vi "VRMSAcqSubVI.vi"(8 "error in (no error)":errorcluster, 11 "Data Cluster in":T1) -> (0 "error out":errorcluster, 2 "RMS value":dbl format="%0.2p", 3 "Data Cluster out":T1)   [LabVIEW 2017]
uses:
  Controls/ShiftRegisterCluster.ctl
  <vilib>/DAQmx/read.llb/DAQmx Read (Analog Wfm 1Chan NSamp).vi
  <vilib>/DAQmx/miscellaneous.llb/DAQmx Fill In Error Info.vi
  <vilib>/measure/madcrms.llb/Basic Averaged DC-RMS for 1 Chan.vi
  <vilib>/measure/NI_MAPro.lvlib
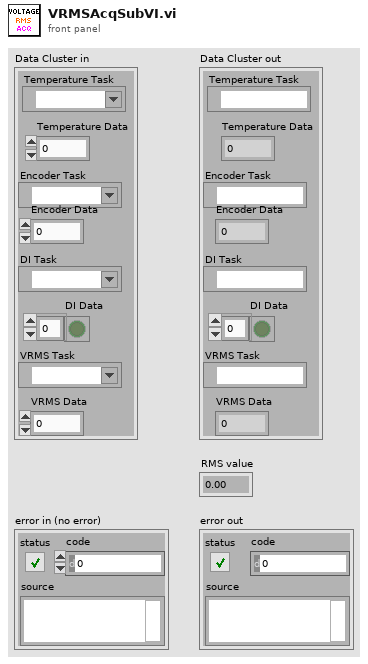
[diagram p1: front panel]
types:
  T1 = typedef "ShiftRegisterCluster.ctl" = cluster{"Temperature Task":refnum<k21>, "Temperature Data":dbl, "Encoder Task":refnum<k21>, "Encoder Data":dbl, "DI Task":refnum<k21>, "DI Data":bool[], "VRMS Task":refnum<k21>, "VRMS Data":dbl}
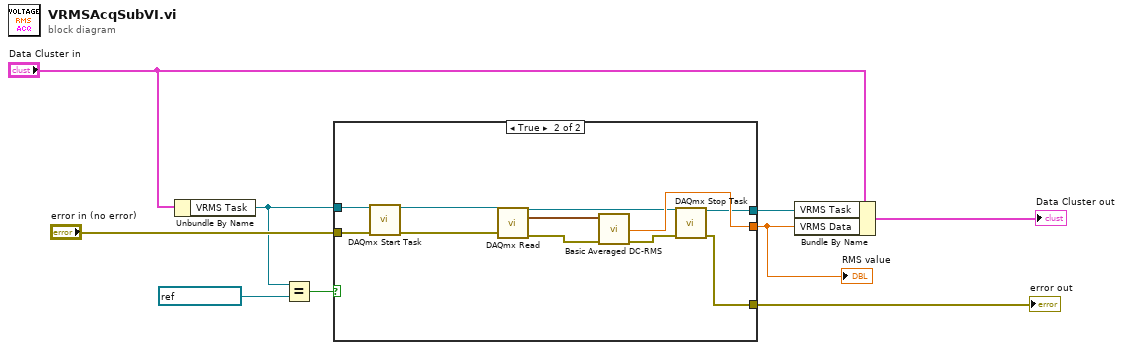
[diagram p0: block diagram]
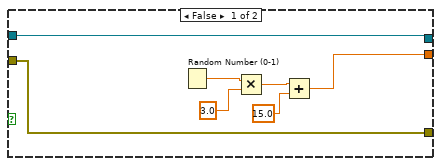
[diagram p2: hidden frame]
diagram:
  n1 = Unbundle By Name("Data Cluster in") -> ("VRMS Task"=w3:refnum<k21>)
  n2 = Equal?(x=w3, y=refnum<k21> "VRMSTask" ("DAQmx Task Name")) -> (x = y?=w1:bool)
  n3 = case shown="True" w1 {
    tunnel: [w11 w27] -> w9
    tunnel: [w16 w23] -> w7
    tunnel: [w10 w22] -> w5
    tunnel: "error in (no error)" -> [w10 w18]
    tunnel: w3 -> [w16 w17]
    frame False {
      n4 = Random Number (0-1)() -> (number: 0 to 1=w15:dbl)
      n5 = Multiply(x=w15, y=3.0) -> (x*y=w13:dbl)
      n6 = Add(x=w13, y=15.0) -> (x+y=w11:dbl)
    }
    frame True {
      n7 = call <vilib>:"DAQmx Start Task.vi"("task/channels in"=w17, "error in"=w18) -> ("task out"=w19:refnum<k21>, "error out"=w20:errorcluster)  [unwired: 12 in]
      n8 = call-poly <vilib>:"DAQmx Read.vi"("task/channels in"=w19, "error in"=w20) -> ("task out"=w21:refnum<k21>, "data"=w24:waveform(dbl), "error out"=w25:errorcluster)  [unwired: 11 in]
      n9 = call-poly <vilib>:"Basic Averaged DC-RMS.vi"("error in (no error)"=w25, "signal in"=w24) -> ("error out"=w26:errorcluster, "RMS value"=w27:dbl)  [unwired: 6 in, 2 out]
      n10 = call <vilib>:"DAQmx Stop Task.vi"("task/channels in"=w21, "error in"=w26) -> ("task out"=w23:refnum<k21>, "error out"=w22:errorcluster)  [unwired: 12 in]
    }
  }
  "RMS value" <- w9
  "error out" <- w5
  n11 = Bundle By Name(cluster="Data Cluster in", "VRMS Task"=w7, "VRMS Data"=w9) -> (→"Data Cluster out":T1)
